vi "Multi Select.vi"(6 "Default":u16, 9 "Selections":u16[](array[numeric]), 11 "Inputs":bool[](array[boolean])) -> (2 "Result":u16)   [LabVIEW 2013]
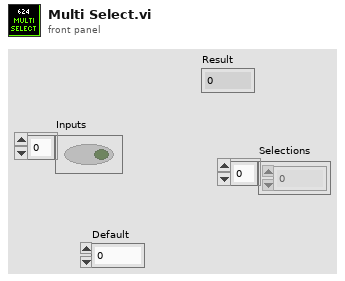
[diagram p1: front panel]
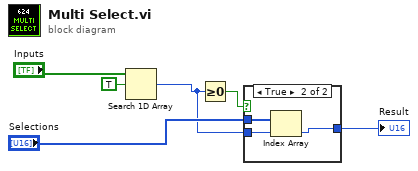
[diagram p0: block diagram]
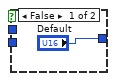
[diagram p2: hidden frame]
diagram:
  n1 = Search 1D Array(1D array="Inputs", element=TRUE) -> (index of element=w2:i32)  [unwired: 1 in]
  n2 = Greater Or Equal To 0?(x=w2) -> (x >= 0?=w3:bool)
  n3 = case shown="True" w3 {
    tunnel: "Selections" -> [_ w10]
    tunnel: w2 -> [_ w9]
    tunnel: ["Default" w8] -> w1
    frame False {
    }
    frame True {
      n4 = Index Array(array=w10, index=w9) -> (element=w8:u16)
    }
  }
  "Result" <- w1
